vi "BotSpeak_AnalogIn.vi"(2 "Bot Settings":T1, 3 "A/D Channel":u8(slide) scale=0.0..10.0) -> (1 "voltage":dbl(knob) scale=-10.0..10.0, 4 "Bot Settings":T1)   [LabVIEW 2014]
doc: "Reads and outputs the \"voltage\" into the specified \"A/D Channel\"."
uses:
  <userlib>/BotSpeak/VIs/Direct/BotSpeak_Control.ctl
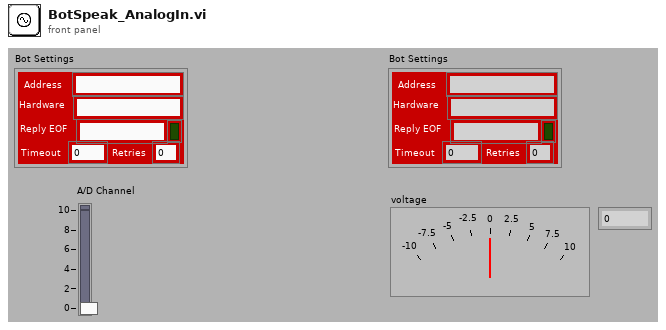
[diagram p1: front panel]
types:
  T1 = typedef "BotSpeak_Control.ctl" = cluster{"Address":string, "Reply EOF":string, "Hardware":string, "Retries":i8, "Timeout":i32, "Open?":bool}
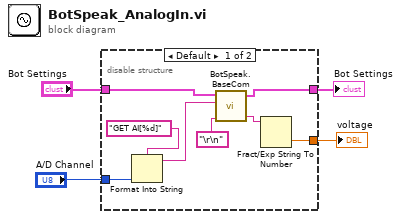
[diagram p0: block diagram]
diagram:
  n1 = disable-structure shown="Default" {
    disable-tunnel: "A/D Channel" -> [w10 _]
    disable-tunnel: [w8 _] -> w3
    disable-tunnel: [w7 _] -> w2
    disable-tunnel: "Bot Settings" -> [w6 _]
    frame condition #0 (active) {
      n2 = Format Into String(format string="GET AI[%d]" ("command"), w10) -> (resulting string=w12:string)  [unwired: 2 in, 1 out]
      n3 = call <userlib>:"BotSpeak.BaseCom.vi"("Termination"="\r\n", "command"=w12, "Bot Settings in"=w6) -> ("response"=w9:string, "Bot Settings out"=w7:T1)  [unwired: 2 in]
      n4 = Fract/Exp String To Number(string=w9) -> (number=w8:dbl)  [unwired: 3 in, 1 out]
    }
    frame condition #1 {
    }
  }
  "voltage" <- w3
  "Bot Settings" <- w2
